vi "Get Page VI.vi"(8 "error in (no error)":errorcluster, 9 "GUID":string, 10 "Item Ref":T1 format="%.0x", 11 "System Explorer Dispatcher Implementation in":refnum<class "System Explorer Dispatcher.lvclass">) -> (0 "error out":errorcluster, 2 "page reference":refnum<vi>, 3 "System Explorer Dispatcher Implementation out":refnum<class "System Explorer Dispatcher.lvclass">)   [LabVIEW 2020, in "Ballard ARINC 429 System Explorer.lvlib" / "Implementation.lvlib" / "System Explorer Dispatcher.lvclass"]
uses:
  System Explorer Dispatcher.lvclass
  <vilib>/NI VeriStand/Custom Device API/Custom Device Item Ref.ctl
  Scripting/Constants.vi
  System Explorer/Pages/Configuration Files.vi
  System Explorer/Pages/Port.vi
  System Explorer/Pages/Channel Specification.vi
  System Explorer/Pages/Parameter.vi
  System Explorer/Pages/Receive Time.vi
  System Explorer/Pages/Word.vi
  System Explorer/Pages/Status.vi
  Implementation.lvlib
  Scripting/Ballard ARINC 429 Scripting.lvlib
  <vilib>/NI VeriStand/Custom Device API/Custom Device API.lvlib
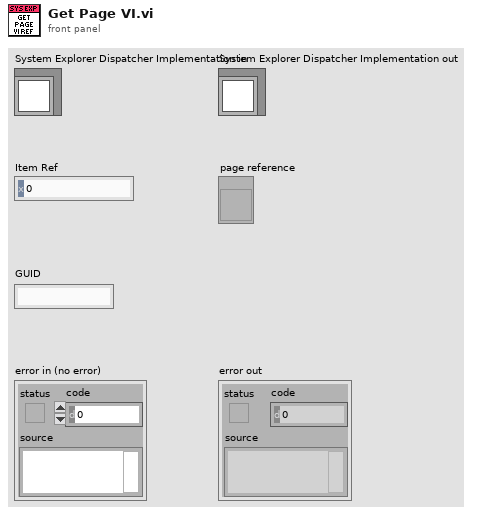
[diagram p1: front panel]
types:
  T1 = typedef "Custom Device API.lvlib/Custom Device Item Ref.ctl" = u64
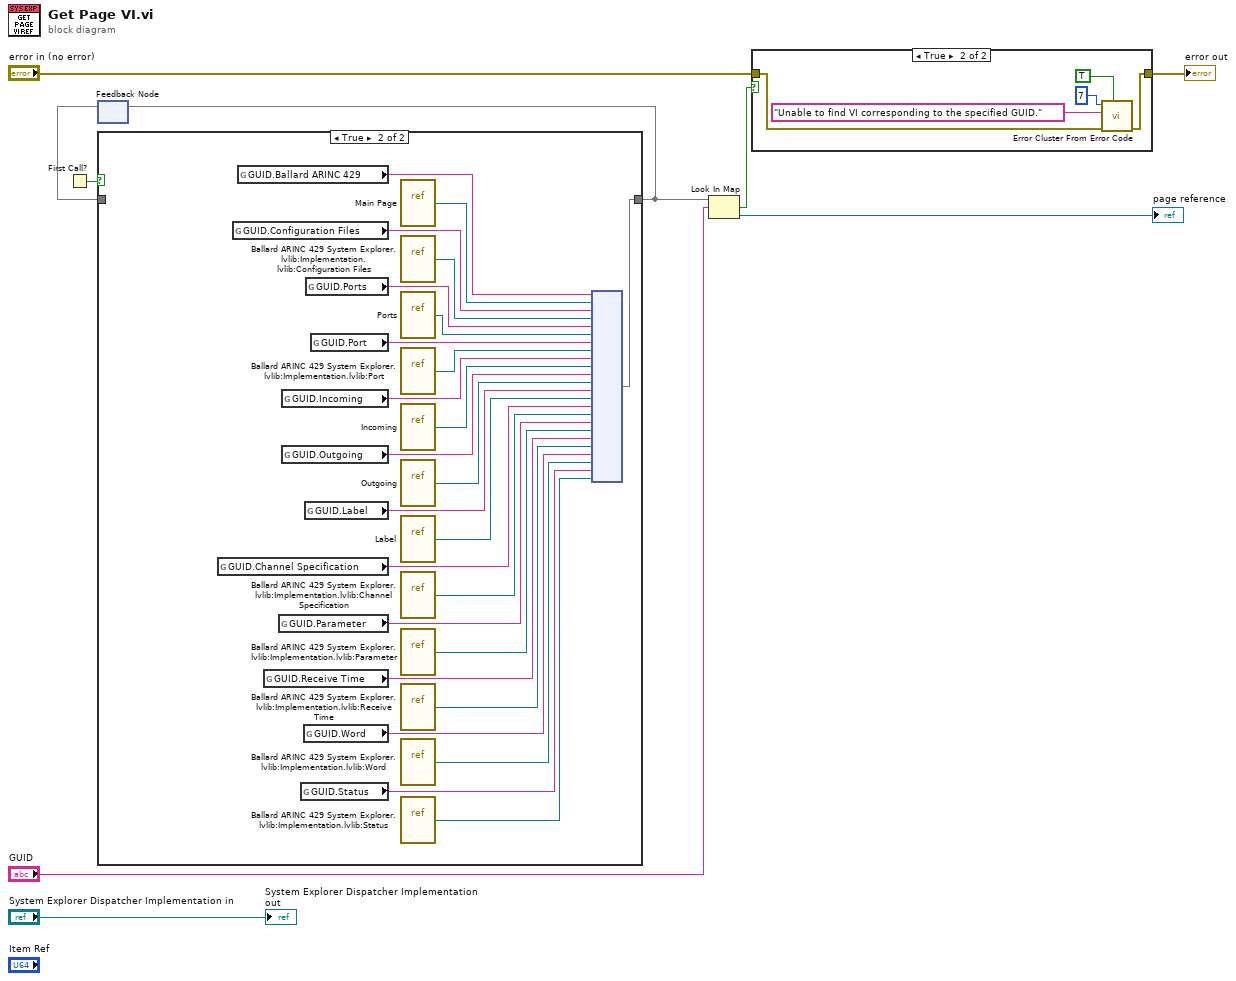
[diagram p0: block diagram]
diagram:
  n1 = First Call?() -> (First Call?: T/F=w8:bool)
  n2 = feedback #1() -> (w7:map{string, refnum<vi>})  [unwired: 1 in]
  n3 = case shown="True" w8 {
    tunnel: [w10 w35] -> w6
    tunnel: w7 -> [w10 _]
    frame False {
    }
    frame True {
      n4 = global read "Constants.vi" "GUID.Channel Specification"() -> (w20:string)
      n5 = global read "Constants.vi" "GUID.Configuration Files"() -> (w31:string)
      n6 = global read "Constants.vi" "GUID.Ballard ARINC 429"() -> (w33:string)
      n7 = global read "Constants.vi" "GUID.Receive Time"() -> (w16:string)
      n8 = global read "Constants.vi" "GUID.Parameter"() -> (w18:string)
      n9 = global read "Constants.vi" "GUID.Incoming"() -> (w26:string)
      n10 = global read "Constants.vi" "GUID.Outgoing"() -> (w24:string)
      n11 = global read "Constants.vi" "GUID.Status"() -> (w12:string)
      n12 = global read "Constants.vi" "GUID.Word"() -> (w14:string)
      n13 = global read "Constants.vi" "GUID.Label"() -> (w22:string)
      n14 = global read "Constants.vi" "GUID.Ports"() -> (w30:string)
      n15 = global read "Constants.vi" "GUID.Port"() -> (w28:string)
      n16 = vi-ref "Main Page.vi"() -> (w34:refnum<vi>)
      n17 = vi-ref "Ballard ARINC 429 System Explorer.lvlib:Implementation.lvlib:Configuration Files.vi"() -> (w32:refnum<vi>)
      n18 = vi-ref "Ports.vi"() -> (w29:refnum<vi>)
      n19 = vi-ref "Ballard ARINC 429 System Explorer.lvlib:Implementation.lvlib:Port.vi"() -> (w27:refnum<vi>)
      n20 = vi-ref "Incoming.vi"() -> (w25:refnum<vi>)
      n21 = vi-ref "Outgoing.vi"() -> (w23:refnum<vi>)
      n22 = vi-ref "Label.vi"() -> (w21:refnum<vi>)
      n23 = vi-ref "Ballard ARINC 429 System Explorer.lvlib:Implementation.lvlib:Channel Specification.vi"() -> (w19:refnum<vi>)
      n24 = vi-ref "Ballard ARINC 429 System Explorer.lvlib:Implementation.lvlib:Parameter.vi"() -> (w17:refnum<vi>)
      n25 = vi-ref "Ballard ARINC 429 System Explorer.lvlib:Implementation.lvlib:Receive Time.vi"() -> (w15:refnum<vi>)
      n26 = vi-ref "Ballard ARINC 429 System Explorer.lvlib:Implementation.lvlib:Word.vi"() -> (w13:refnum<vi>)
      n27 = vi-ref "Ballard ARINC 429 System Explorer.lvlib:Implementation.lvlib:Status.vi"() -> (w11:refnum<vi>)
      n28 = node(w33, w34, w31, w32, w30, w29, w28, w27, w26, w25, w24, w23, w22, w21, w20, w19, w18, w17, w16, w15, w14, w13, w12, w11) -> (w35:map{string, refnum<vi>})
    }
  }
  n29 = feedback-in #1(w6) -> ()
  n30 = Look In Map(map=w6, key="GUID") -> (key not found?=w4:bool, value=→"page reference":refnum<vi>)  [unwired: 1 in]
  n31 = case shown="True" w4 {
    tunnel: [w36 w38] -> w3
    tunnel: "error in (no error)" -> [w36 w37]
    frame False {
    }
    frame True {
      n32 = call <vilib>:"Error Cluster From Error Code.vi"("show call chain? (False)"=TRUE, "error in (no error)"=w37, "error message (\"\")"="Unable to find VI corresponding to the specified GUID." ("error message (\"\")"), "error code (0)"=7) -> ("error out"=w38:errorcluster)  [unwired: 5 in]
    }
  }
  "error out" <- w3
  "System Explorer Dispatcher Implementation out" <- "System Explorer Dispatcher Implementation in"
